vi "Set_Env_Var.vi"(6 "Value":string, 7 "Environment Variable Name":string) -> ()   [LabVIEW 2020]
uses:
  kernel32.dll
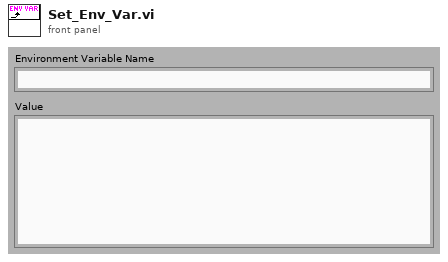
[diagram p1: front panel]
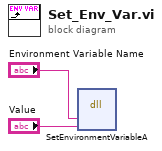
[diagram p0: block diagram]
diagram:
  n1 = dll-call lib="kernel32.dll" fn="SetEnvironmentVariableA"("EnvVarName"="Environment Variable Name", "Value"="Value") -> ()  [unwired: 6 in, 2 out]
